vi "1A VBattSense FPGA.vi"() -> ()   [LabVIEW 2011]
uses:
  <vilib>/rvi/eio/common/nirviEmuTemplateMethod_errors.vi
  <vilib>/eio/EIONode/EIONode.xnode
panel:
  in  "stop VBatt Sense":bool
  out "vBatt*0.3":u8
  out "VBatt bit7":bool
  out "VBatt bit6":bool
  out "VBatt bit5":bool
  out "VBatt bit4":bool
  out "VBatt bit3":bool
  out "VBatt bit2":bool
  out "VBatt bit1":bool
  out "VBatt bit0":bool
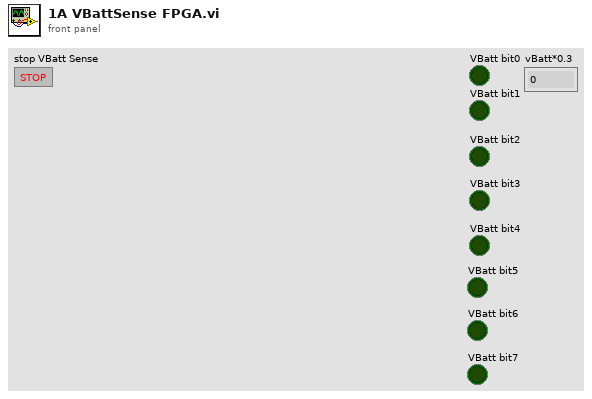
[diagram p1: front panel]
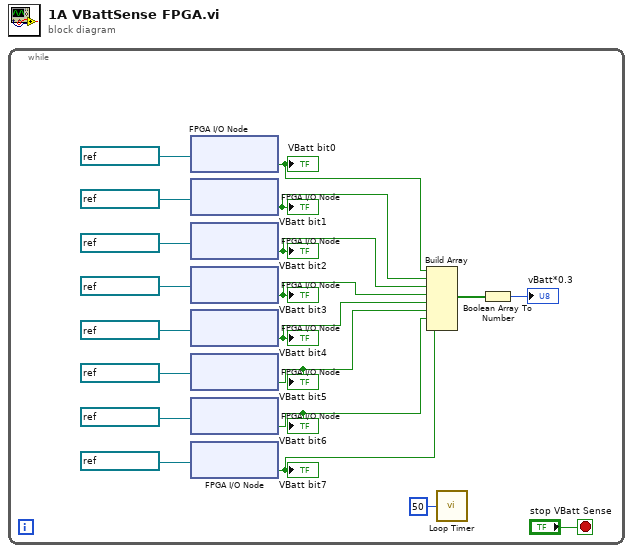
[diagram p0: block diagram]
diagram:
  n1 = while {
    stop <- "stop VBatt Sense" stop-if-true
    n2 = xnode "FPGA I/O Node"("FPGA I/O In"=refnum<k21> "VBatt bit0") -> ("I/O Item"=w5:bool)  [unwired: 1 out]
    "VBatt bit0" <- w5
    n3 = xnode "FPGA I/O Node"("FPGA I/O In"=refnum<k21> "VBatt bit0") -> ("I/O Item"=w6:bool)  [unwired: 1 out]
    "VBatt bit1" <- w6
    n4 = xnode "FPGA I/O Node"("FPGA I/O In"=refnum<k21> "VBatt bit0") -> ("I/O Item"=w7:bool)  [unwired: 1 out]
    "VBatt bit2" <- w7
    n5 = xnode "FPGA I/O Node"("FPGA I/O In"=refnum<k21> "VBatt bit0") -> ("I/O Item"=w8:bool)  [unwired: 1 out]
    "VBatt bit3" <- w8
    n6 = xnode "FPGA I/O Node"("FPGA I/O In"=refnum<k21> "VBatt bit0") -> ("I/O Item"=w9:bool)  [unwired: 1 out]
    "VBatt bit4" <- w9
    n7 = xnode "FPGA I/O Node"("FPGA I/O In"=refnum<k21> "VBatt bit0") -> ("I/O Item"=w10:bool)  [unwired: 1 out]
    "VBatt bit5" <- w10
    n8 = xnode "FPGA I/O Node"("FPGA I/O In"=refnum<k21> "VBatt bit0") -> ("I/O Item"=w11:bool)  [unwired: 1 out]
    "VBatt bit6" <- w11
    n9 = xnode "FPGA I/O Node"("FPGA I/O In"=refnum<k21> "VBatt bit7") -> ("I/O Item"=w12:bool)  [unwired: 1 out]
    "VBatt bit7" <- w12
    n10 = Build Array(w5, w6, w7, w8, w9, w10, w11, w12) -> (w4:bool[])
    n11 = call "Loop Timer"("Count(mSec)"=u32 50) -> ()  [unwired: 1 out]
    n12 = Boolean Array To Number(Boolean array=w4) -> (number=→"vBatt*0.3":u8)
  }
